vi "StopAndWaitForIdle.vi"(11 "error in (no error)":errorcluster) -> (3 "error out":errorcluster, 5 "Changed?":bool)   [LabVIEW 2018, in "AcPwrModule.lvlib"]
uses:
  AcPwrModule.lvlib
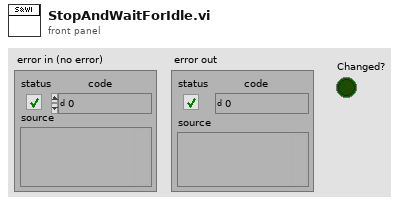
[diagram p1: front panel]
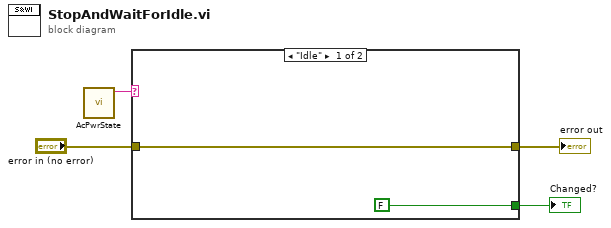
[diagram p0: block diagram]
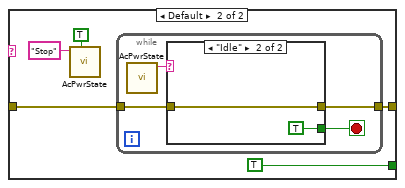
[diagram p2: hidden frame]
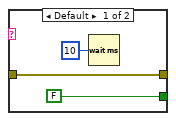
[diagram p3: hidden frame]
diagram:
  n1 = call "AcPwrState.vi"() -> ("strngStateOut"=w4:string)  [unwired: 11 in]
  n2 = case shown="\"Idle\"" w4 {
    tunnel: [w5 w11] -> w1
    tunnel: [FALSE TRUE] -> w2
    tunnel: "error in (no error)" -> [w5 w7]
    frame "Idle" {
    }
    frame Default {
      n3 = call "AcPwrState.vi"("Set"=TRUE, "strngStateIn"="Stop") -> ()  [unwired: 9 in, 1 out]
      n4 = while {
        tunnel: w7 -> [w14]
        tunnel: [w13] -> w11
        stop <- w12 stop-if-true
        n5 = call "AcPwrState.vi"() -> ("strngStateOut"=w15:string)  [unwired: 11 in]
        n6 = case shown="\"Idle\"" w15 {
          tunnel: w14 -> [w18 w20]
          tunnel: [w18 w20] -> w13
          tunnel: [FALSE TRUE] -> w12
          frame Default {
            n7 = Wait (ms)(milliseconds to wait=u32 10) -> ()  [unwired: 1 out]
          }
          frame "Idle" {
          }
        }
      }
    }
  }
  "Changed?" <- w2
  "error out" <- w1
